vi "CRYSet Serial Editor Front Panel.vi"(11 "Vi Ref":refnum<vi>) -> ()   [LabVIEW 2013]
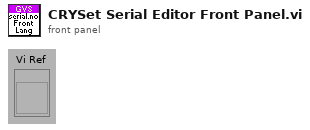
[diagram p1: front panel]
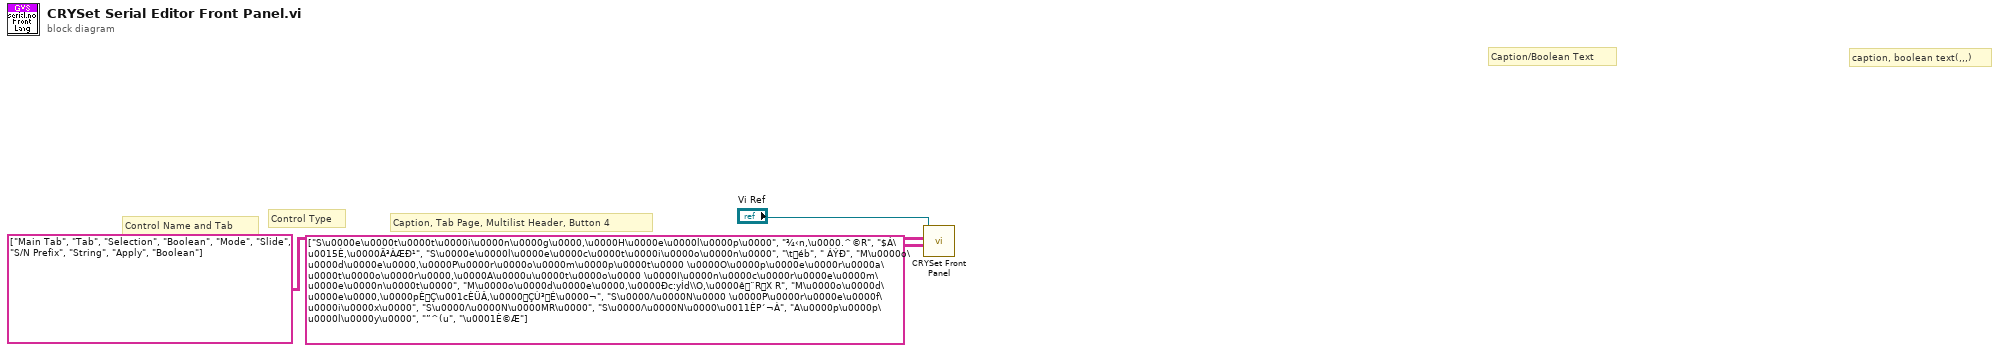
[diagram p0: block diagram]
diagram:
  # "Caption, Tab Page, Multilist Header, Button 4"
  # "Control Type"
  # "Control Name and Tab"
  # "caption, boolean text(,,,)"
  # "Caption/Boolean Text"
  n1 = call "CRYSet Front Panel.vi"("Caption(Boolean Text)"=string[][] [["S\u0000e\u0000t\u0000t\u0000i\u0000n\u0000g\u0000,\u0000H\u0000e\u0000l\u0000p\u0000", "¾‹n,\u0000.^©R", "$Á\u0015È,\u0000Ä³ÀÆÐ¹"], ["S\u0000e\u0000l\u0000e\u0000c\u0000t\u0000i\u0000o\u0000n\u0000", "\téb", " ÁÝÐ"], ["M\u0000o\u0000d\u0000e\u0000,\u0000P\u0000r\u0000o\u0000m\u0000p\u0000t\u0000 \u0000O\u0000p\u0000e\u0000r\u0000a\u0000t\u0000o\u0000r\u0000,\u0000A\u0000u\u0000t\u0000o\u0000 \u0000I\u0000n\u0000c\u0000r\u0000e\u0000m\u0000e\u0000n\u0000t\u0000", "M\u0000o\u0000d\u0000e\u0000,\u0000Ðc:yÍd\\O,\u0000ê¨RX R", "M\u0000o\u0000d\u0000e\u0000,\u0000pÈÇ\u001cÈÜÂ,\u0000ÇÙ³É\u0000¬"], ["S\u0000/\u0000N\u0000 \u0000P\u0000r\u0000e\u0000f\u0000i\u0000x\u0000", "S\u0000/\u0000N\u0000MR\u0000", "S\u0000/\u0000N\u0000\u0011ÈP´¬À"], ["A\u0000p\u0000p\u0000l\u0000y\u0000", "”^(u", "\u0001È©Æ"]], "Control ID and Type(Label Name, Type)"=string[][] [["Main Tab", "Tab"], ["Selection", "Boolean"], ["Mode", "Slide"], ["S/N Prefix", "String"], ["Apply", "Boolean"]], "Vi Ref"="Vi Ref") -> ()  [unwired: 9 in]
